vi "Set Discrete Sweep Attributes.vi"(4 "Measurement Time":dbl, 5 "Spacing":u16, 6 "Measurement Cycles":dbl, 7 "Steps":i32, 9 "stop":dbl=10000.0 format="%.2f", 10 "start":dbl=10.0 format="%.2f", 11 "Display State Attributes in":variant) -> (2 "name":string="DiscreteSweepInfo", 3 "Display State Attributes out":variant)   [LabVIEW 2017, in "Test Signal Configuration.xctl"]
uses:
  <vilib>/addons/_XControls/Function Generator Configuration/Test Signal Configuration.xctl
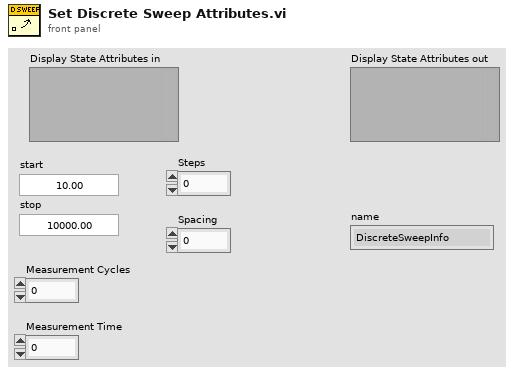
[diagram p1: front panel]
types:
  T1 = typedef "Test Signal Configuration.xctl/signal type.ctl" = enum32{"None", "Tone", "Multitone", "Discrete Sweep", "Continuous Sweep", "Noise"}
  T2 = cluster{"Signal":cluster{"Sample Rate":cluster{"name":string, "default":dbl}, "Signal Type":cluster{"name":string, "signal type":T1}, "Amplitude":cluster{"name":string, "default":dbl}, "Offset":cluster{"name":string, "default":dbl}}, "Function":cluster{"Info":cluster{"name":string, "default":variant}, "Type":cluster{"name":string, "default":u16}, "Frequency":cluster{"name":string, "default":dbl}, "Phase":cluster{"name":string, "default":dbl}}, "Continuous Sweep":cluster{"Info":cluster{"name":string, "default":variant}, "Start":cluster{"name":string, "default":dbl}, "Stop":cluster{"name":string, "default":dbl}, "Duration":cluster{"name":string, "default":dbl}, "Profile":cluster{"name":string, "default":enum16{"Linear", "Logarithmic"}}}, "Discrete Sweep":cluster{"Info":cluster{"name":string, "default":variant}, "Start":cluster{"name":string, "default":dbl}, "Stop":cluster{"name":string, "default":dbl}, "Cycles":cluster{"name":string, "default":dbl}, "Time":cluster{"name":string, "default":dbl}, "Spacing":cluster{"name":string, "default":enum16{"Linear", "Logarithmic"}}, "Steps":cluster{"name":string, "default":i32}}, "Multitone":cluster{"Info":cluster{"name":string, "multitone info":cluster{"frequency":dbl, "amplitude":dbl, "phase":dbl}[]}}, "Noise":cluster{"Info":cluster{"name":string, "default":variant}, "Type":cluster{"name":string, "default":u16}, "Amplitude PDF":cluster{"name":string, "default":enum16{"Gaussian", "Rectangular", "Triangular"}}, "Level":cluster{"name":string, "default":dbl}, "Seed":cluster{"name":string, "default":i32}}, "Configuration":cluster{"Min Frequency":cluster{"name":string, "default":dbl}, "Max Frequency":cluster{"name":string, "default":dbl}, "Max Amplitude":cluster{"name":string, "default":dbl}}}
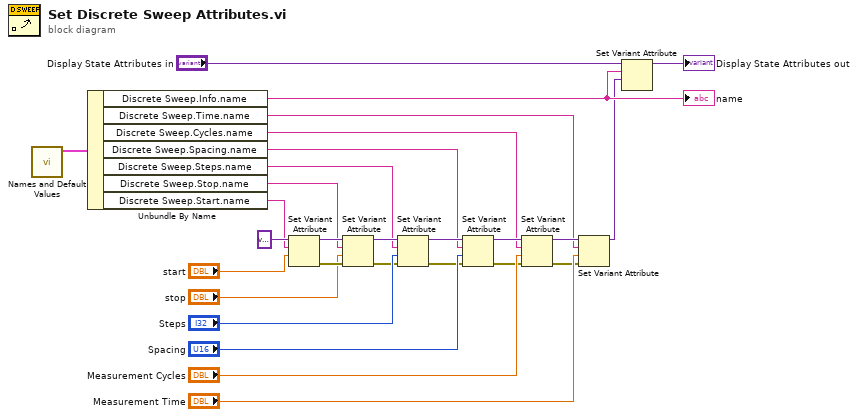
[diagram p0: block diagram]
diagram:
  n1 = call <vilib>:"Names and Default Values.vi"() -> ("Names and Default Values"=w13:T2)  [unwired: 11 in]
  n2 = Unbundle By Name(w13) -> ("Discrete Sweep.Info.name"=w4:string, "Discrete Sweep.Time.name"=w7:string, "Discrete Sweep.Cycles.name"=w8:string, "Discrete Sweep.Spacing.name"=w9:string, "Discrete Sweep.Steps.name"=w10:string, "Discrete Sweep.Stop.name"=w11:string, "Discrete Sweep.Start.name"=w12:string)
  "name" <- w4
  n3 = Set Variant Attribute(Variant=variant ("variant"), name=w12, value="start") -> (Variant out=w16:variant, error out=w15:errorcluster)  [unwired: 1 in, 1 out]
  n4 = Set Variant Attribute(Variant=w16, name=w11, value="stop", error in=w15) -> (Variant out=w20:variant, error out=w19:errorcluster)  [unwired: 1 out]
  n5 = Set Variant Attribute(Variant=w20, name=w10, value="Steps", error in=w19) -> (Variant out=w18:variant, error out=w17:errorcluster)  [unwired: 1 out]
  n6 = Set Variant Attribute(Variant=w18, name=w9, value="Spacing", error in=w17) -> (Variant out=w22:variant, error out=w21:errorcluster)  [unwired: 1 out]
  n7 = Set Variant Attribute(Variant=w22, name=w8, value="Measurement Cycles", error in=w21) -> (Variant out=w24:variant, error out=w23:errorcluster)  [unwired: 1 out]
  n8 = Set Variant Attribute(Variant=w24, name=w7, value="Measurement Time", error in=w23) -> (Variant out=w3:variant)  [unwired: 2 out]
  n9 = Set Variant Attribute(Variant="Display State Attributes in", name=w4, value=w3) -> (Variant out=→"Display State Attributes out":variant)  [unwired: 1 in, 2 out]
